vi "Mouse Down_User Layers.vi"(7 "Shift":bool, 8 "error in":errorcluster, 9 "Ctrl":bool, 10 "CtlRef":refnum<vi>, 11 "Data in":T1={"Class"={"Ants"=refnum, "Layer"=refnum, "Templates"=refnum, "Icon"=refnum, "Glyph"=refnum, "Settings"=refnum, "Tools"=refnum}, "Ref"={"Add Layer"=refnum, "Remove Layer"=refnum, "Line Text"=[], "Body Text Spec"=refnum, "DNL_Font"=refnum, "glyph path str"=refnum, "templates path str"=refnum, "Arrow Up"=refnum, "Arrow Down"=refnum, "IE VI Ref"=refnum, "Glyphs tree"=refnum, "Templates tree"=refnum, "Layer Icon Text"=refnum, "Layer Template"=refnum, "Body Text"=refnum, "Search Templates"=refnum, "TextMarker"=refnum, "Tab Control"=refnum, "Search Glyphs"=refnum, "Line Color"=refnum, "DNL_Glyphs []"=refnum, "Fill Color"=refnum, "Tools"=refnum, "Icon"=refnum, "Preview"=refnum, "Ants"=refnum, "Terminals"=refnum, "menu reference"=refnum, "LayerNames"=[], "GlyphLoadAnimation"=refnum, "TemplateLoadAnimation"=refnum, "refreshGlyphs"=refnum, "refreshTemplates"=refnum}, "Support"={"AntsRect"={"left"=0, "top"=0, "right"=0, "bottom"=0}, "Mouse Move Coords"={"Horizontal"=0, "Vertical"=0}, "Mouse Down Coords"={"Horizontal"=0, "Vertical"=0}, "Temp Coord"={"Horizontal"=0, "Vertical"=0}, "Action"=enum."Default", "Edge Color"=4914962, "Fill Color"=16860, "Mouse Down?"=FALSE, "Draft Mode?"=FALSE, "Temp Icon"=bytes[3102], "CTRL Pressed"=FALSE, "Move Selection?"=FALSE, "AntsRect Orig"={"left"=0, "top"=0, "right"=0, "bottom"=0}, "Text"="", "TM Set?"=FALSE, "Mouse inside icon?"=FALSE, "Tool (old value)"=0, "Pencil Move Color"=0, "Swap Colors?"=FALSE, "Shift pressed?"=FALSE}}) -> (0 "error out":errorcluster, 3 "Data out":T1={"Class"={"Ants"=refnum, "Layer"=refnum, "Templates"=refnum, "Icon"=refnum, "Glyph"=refnum, "Settings"=refnum, "Tools"=refnum}, "Ref"={"Add Layer"=refnum, "Remove Layer"=refnum, "Line Text"=[], "Body Text Spec"=refnum, "DNL_Font"=refnum, "glyph path str"=refnum, "templates path str"=refnum, "Arrow Up"=refnum, "Arrow Down"=refnum, "IE VI Ref"=refnum, "Glyphs tree"=refnum, "Templates tree"=refnum, "Layer Icon Text"=refnum, "Layer Template"=refnum, "Body Text"=refnum, "Search Templates"=refnum, "TextMarker"=refnum, "Tab Control"=refnum, "Search Glyphs"=refnum, "Line Color"=refnum, "DNL_Glyphs []"=refnum, "Fill Color"=refnum, "Tools"=refnum, "Icon"=refnum, "Preview"=refnum, "Ants"=refnum, "Terminals"=refnum, "menu reference"=refnum, "LayerNames"=[], "GlyphLoadAnimation"=refnum, "TemplateLoadAnimation"=refnum, "refreshGlyphs"=refnum, "refreshTemplates"=refnum}, "Support"={"AntsRect"={"left"=0, "top"=0, "right"=0, "bottom"=0}, "Mouse Move Coords"={"Horizontal"=0, "Vertical"=0}, "Mouse Down Coords"={"Horizontal"=0, "Vertical"=0}, "Temp Coord"={"Horizontal"=0, "Vertical"=0}, "Action"=enum."Default", "Edge Color"=4914962, "Fill Color"=16860, "Mouse Down?"=FALSE, "Draft Mode?"=FALSE, "Temp Icon"=bytes[3102], "CTRL Pressed"=FALSE, "Move Selection?"=FALSE, "AntsRect Orig"={"left"=0, "top"=0, "right"=0, "bottom"=0}, "Text"="", "TM Set?"=FALSE, "Mouse inside icon?"=FALSE, "Tool (old value)"=0, "Pencil Move Color"=0, "Swap Colors?"=FALSE, "Shift pressed?"=FALSE}})   [LabVIEW 2020]
uses:
  Class/Ants/Ants.lvclass
  Class/FakedArray/FakedArray.lvclass
  vi.lib/LabVIEW Icon API/lv_icon/Classes/Icon/Icon.lvclass
  Class/Icon Library/Glyph.lvclass
  Class/Settings/Settings.lvclass
  Class/Tools/Tools Paint.lvclass
  <vilib>/Utility/miscctls.llb/LVPoint32TypeDef.ctl
  Controls/SupportClass_Action.ctl
  vi.lib/LabVIEW Icon API/lv_icon/Controls/IEColor.ctl
  Controls/SupportClass.ctl
  Controls/References Cluster.ctl
  vi.lib/LabVIEW Icon API/lv_icon/lv_icon.lvlib
  Controls/IE Classes.ctl
  Controls/Global Data.ctl
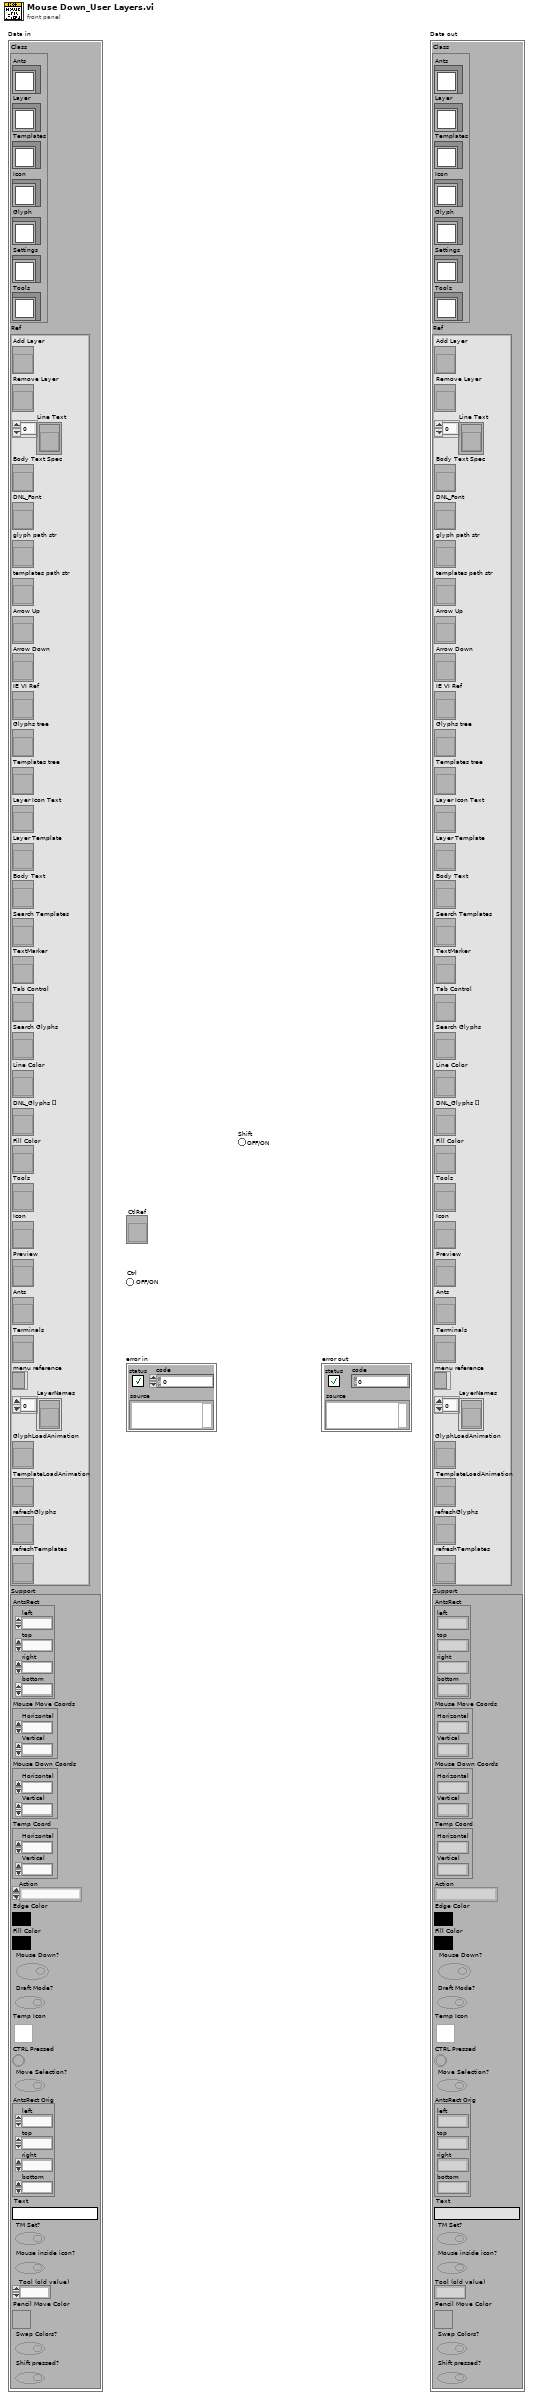
[diagram p1: front panel]
types:
  T1 = typedef "lv_icon.lvlib/Global Data.ctl" = cluster{"Class":T2, "Ref":T3, "Support":T4}
  T2 = typedef "IE Classes.ctl" = cluster{"Ants":refnum<class "Ants.lvclass">, "Layer":refnum<class "FakedArray.lvclass">, "Templates":refnum<class "FakedArray.lvclass">, "Icon":refnum<class "Icon.lvclass">, "Glyph":refnum<class "Glyph.lvclass">, "Settings":refnum<class "Settings.lvclass">, "Tools":refnum<class "Tools Paint.lvclass">}
  T3 = typedef "lv_icon.lvlib/References Cluster.ctl" = cluster{"Add Layer":refnum<vi>, "Remove Layer":refnum<vi>, "Line Text":refnum<vi>[], "Body Text Spec":refnum<vi>, "DNL_Font":refnum<vi>, "glyph path str":refnum<vi>, "templates path str":refnum<vi>, "Arrow Up":refnum<vi>, "Arrow Down":refnum<vi>, "IE VI Ref":refnum<vi>, "Glyphs tree":refnum<vi>, "Templates tree":refnum<vi>, "Layer Icon Text":refnum<vi>, "Layer Template":refnum<vi>, "Body Text":refnum<vi>, "Search Templates":refnum<vi>, "TextMarker":refnum<vi>, "Tab Control":refnum<vi>, "Search Glyphs":refnum<vi>, "Line Color":refnum<vi>, "DNL_Glyphs []":refnum<vi>, "Fill Color":refnum<vi>, "Tools":refnum<vi>, "Icon":refnum<vi>, "Preview":refnum<vi>, "Ants":refnum<vi>, "Terminals":refnum<vi>, "menu reference":refnum<k9>, "LayerNames":refnum<vi>[], "GlyphLoadAnimation":refnum<vi>, "TemplateLoadAnimation":refnum<vi>, "refreshGlyphs":refnum<vi>, "refreshTemplates":refnum<vi>}
  T4 = typedef "SupportClass.ctl" = cluster{"AntsRect":cluster{"left":i16, "top":i16, "right":i16, "bottom":i16}, "Mouse Move Coords":T5, "Mouse Down Coords":T5, "Temp Coord":T5, "Action":T6, "Edge Color":T7, "Fill Color":T7, "Mouse Down?":bool, "Draft Mode?":bool, "Temp Icon":picture, "CTRL Pressed":bool, "Move Selection?":bool, "AntsRect Orig":cluster{"left":i16, "top":i16, "right":i16, "bottom":i16}, "Text":string, "TM Set?":bool, "Mouse inside icon?":bool, "Tool (old value)":u32, "Pencil Move Color":u32, "Swap Colors?":bool, "Shift pressed?":bool}
  T5 = typedef "LVPoint32TypeDef.ctl" = cluster{"Horizontal":i32, "Vertical":i32}
  T6 = typedef "SupportClass_Action.ctl" = enum16{"Default", "Move Selection", "Glyph Library", "Tool"}
  T7 = typedef "IEColor.ctl" = u32
  T8 = cluster{"left":i16, "top":i16, "right":i16, "bottom":i16}
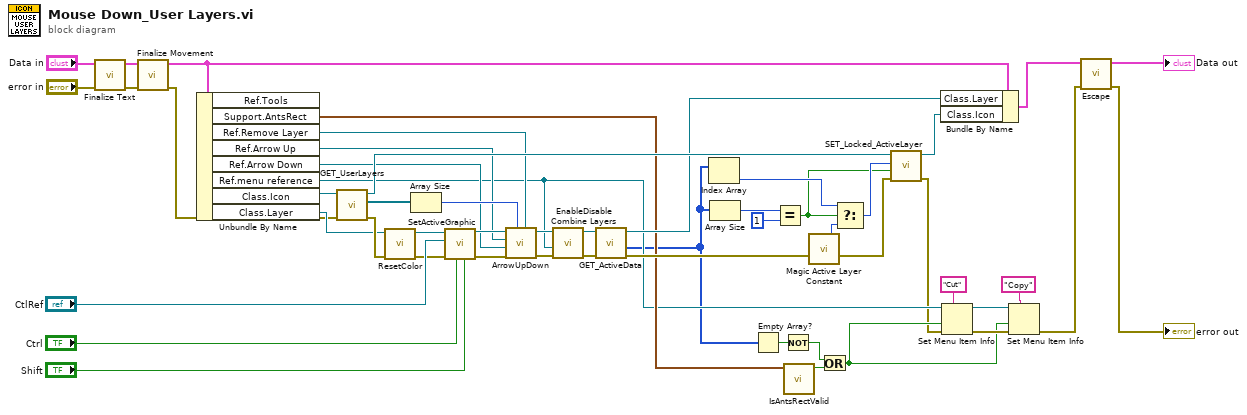
[diagram p0: block diagram]
diagram:
  n1 = call "Finalize Text.vi"("error in (no error)"="error in", "Data in"="Data in") -> ("error out"=w13:errorcluster, "Data out"=w10:T1)  [unwired: 8 out]
  n2 = call "Finalize Movement.vi"("error in (no error)"=w13, "Data in"=w10) -> ("error out"=w8:errorcluster, "Data out"=w11:T1)  [unwired: 1 in, 7 out]
  n3 = Unbundle By Name(w11) -> ("Support.AntsRect"=w18:T8, "Ref.Remove Layer"=w24:refnum<vi>, "Ref.Arrow Up"=w25:refnum<vi>, "Ref.Arrow Down"=w26:refnum<vi>, "Ref.menu reference"=w17:refnum<k9>, "Class.Icon"=w31:refnum<class "Icon.lvclass">, "Class.Layer"=w30:refnum<class "FakedArray.lvclass">)  [unwired: 1 out]
  n4 = call-dynamic "GET_UserLayers.vi"("error in (no error)"=w8, "Icon.lvclass in"=w31) -> ("error out"=w49:errorcluster, "All Layers"=w50:refnum<class "Layer.lvclass">[], "Icon.lvclass out"=w40:refnum<class "Icon.lvclass">)  [unwired: 7 out]
  n5 = call "ResetColor.vi"("error in (no error)"=w49, "FakedArray in"=w30) -> ("error out"=w44:errorcluster, "FakedArray out"=w43:refnum<class "FakedArray.lvclass">)  [unwired: 8 out]
  n6 = Array Size(array=w50) -> (size(s)=w51:i32)
  n7 = call-dynamic "SetActiveGraphic.vi"("Shift"="Shift", "CTRL?"="Ctrl", "error in (no error)"=w44, "Ctl Refnum"="CtlRef", "FakedArray in"=w43) -> ("error out"=w47:errorcluster, "FakedArray out"=w48:refnum<class "FakedArray.lvclass">)  [unwired: 1 in, 4 out]
  n8 = call "ArrowUpDown.vi"("Remove Layer"=w24, "# Layers"=w51, "error in (no error)"=w47, "Arrow Down"=w26, "Arrow Up"=w25, "FakedArray in"=w48) -> ("error out"=w42:errorcluster, "FakedArray out"=w41:refnum<class "FakedArray.lvclass">)  [unwired: 4 out]
  n9 = call "EnableDisable Combine Layers.vi"("error in"=w42, "menu reference"=w17, "Layers Cluster"=w41) -> ("error out"=w39:errorcluster, "FakedArray out"=w38:refnum<class "FakedArray.lvclass">)  [unwired: 1 in, 6 out]
  n10 = call-dynamic "GET_ActiveData.vi"("error in (no error)"=w39, "FakedArray in"=w38) -> ("error out"=w27:errorcluster, "Active Data []"=w7:i32[], "FakedArray out"=w29:refnum<class "FakedArray.lvclass">)  [unwired: 7 out]
  n11 = Index Array(array=w7) -> (element=w35:i32)  [unwired: 1 in]
  n12 = Array Size(array=w7) -> (size(s)=w37:i32)
  n13 = Empty Array?(array=w7) -> (empty?=w6:bool)
  n14 = Equal?(x=w37, y=1) -> (x = y?=w15:bool)
  n15 = Not(x=w6) -> (.not. x?=w5:bool)
  n16 = call "IsAntsRectValid.vi"("AntsRect"=w18) -> ("Valid?"=w16:bool)  [unwired: 10 out]
  n17 = call "Magic Active Layer Constant.vi"() -> ("Magic Constant"=w34:i32)  [unwired: 19 out]
  n18 = Or(x=w5, y=w16) -> (x .or. y?=w19:bool)
  n19 = Select(t=w35, s=w15, f=w34) -> (s? t:f=w33:i32)
  n20 = call-dynamic "SET_Locked_ActiveLayer.vi"("error in (no error)"=w27, "Layers Locked?"=w15, "Active Layer"=w33, "Icon.lvclass in"=w40) -> ("error out"=w14:errorcluster, "Icon.lvclass out"=w28:refnum<class "Icon.lvclass">)  [unwired: 6 out]
  n21 = Bundle By Name(cluster=w11, "Class.Layer"=w29, "Class.Icon"=w28) -> (w4:T1)
  n22 = Set Menu Item Info(7:"Cut" ("item tag"), 8:w14, 9:w19, 11:w17) -> (0:w23:errorcluster, 3:w21:refnum<k9>)  [unwired: 3 out]
  n23 = Set Menu Item Info(7:"Copy" ("item tag"), 8:w23, 9:w19, 11:w21) -> (0:w2:errorcluster)  [unwired: 4 out]
  n24 = call "Escape.vi"("error in"=w2, "Data in"=w4) -> ("error out"=→"error out":errorcluster, "Data out"=→"Data out":T1)  [unwired: 2 in, 6 out]
